vi "Write Measurement.lvclass.vi"(10 "Measurement Actor.lvlib:Measurement.lvclass":refnum<class "Measurement.lvclass">, 11 "Add Available Measurement Msg in":refnum<class "Add Available Measurement Msg.lvclass">) -> (3 "Add Available Measurement Msg out":refnum<class "Add Available Measurement Msg.lvclass">)   [LabVIEW 2026, in "Controller Actor.lvlib" / "Add Available Measurement Msg.lvclass"]
uses:
  Add Available Measurement Msg.lvclass
  Add Available Measurement Msg.lvclass/Add Available Measurement Msg.ctl
  Measurement Actor/Measurement.lvclass
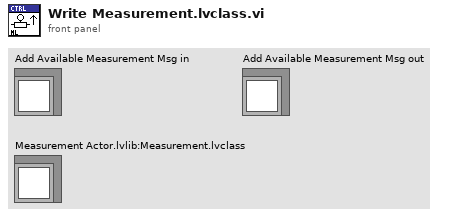
[diagram p1: front panel]
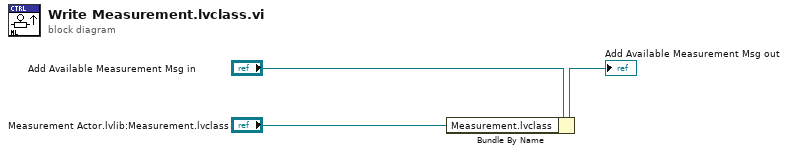
[diagram p0: block diagram]
diagram:
  n1 = Bundle By Name(cluster="Add Available Measurement Msg in", "Measurement.lvclass"="Measurement Actor.lvlib:Measurement.lvclass") -> (→"Add Available Measurement Msg out":refnum<class "Add Available Measurement Msg.lvclass">)
